vi "ChannelsHasWaveforms.vi"(11 "channels":T1[](array[typedef])) -> (2 "has waveforms":bool)   [LabVIEW 2017, in "DeviceModelHelpers.lvlib"]
doc: "Checks whether a channel has waveforms."
uses:
  <vilib>/addons/InsightCM/Utilities/DeviceModelHelpers/DeviceModelHelpers.lvlib
  <vilib>/addons/InsightCM/MessageBus/Base/controls/R2_Channel.ctl
  <vilib>/addons/InsightCM/MessageBus/Base/controls/KeyValuePair.ctl
  <vilib>/addons/InsightCM/MessageBus/Base/controls/Metric.ctl
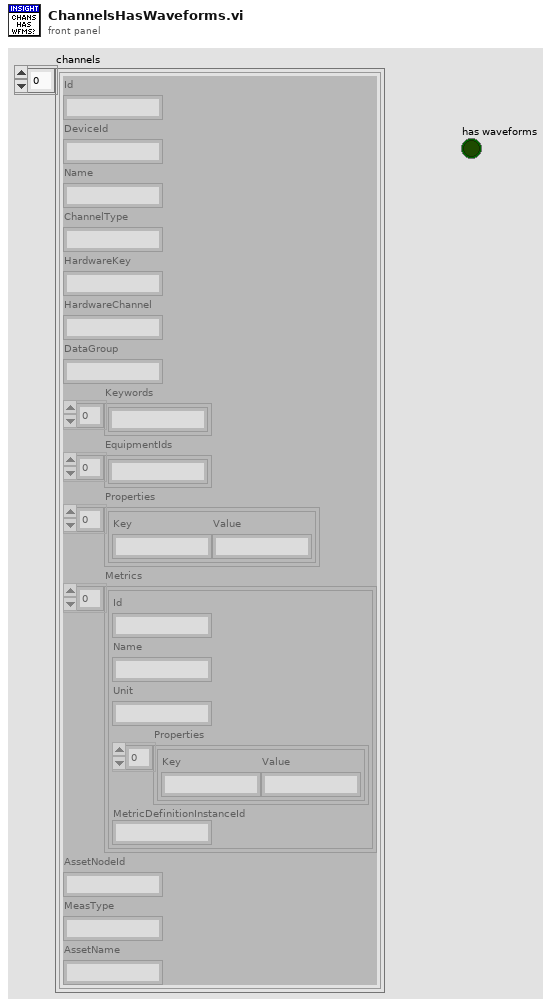
[diagram p1: front panel]
types:
  T1 = typedef "R2_Channel.ctl" = cluster{"Id":string, "DeviceId":string, "Name":string, "ChannelType":string, "HardwareKey":string, "HardwareChannel":string, "DataGroup":string, "Keywords":string[], "EquipmentIds":string[], "Properties":T2[], "Metrics":T3[], "AssetNodeId":string, "MeasType":string, "AssetName":string}
  T2 = typedef "KeyValuePair.ctl" = cluster{"Key":string, "Value":string}
  T3 = typedef "Metric.ctl" = cluster{"Id":string, "Name":string, "Unit":string, "Properties":T2[], "MetricDefinitionInstanceId":string}
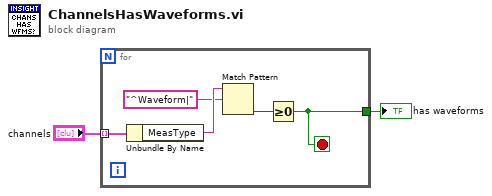
[diagram p0: block diagram]
diagram:
  n1 = for {
    tunnel: "channels" -> [w7] mode=indexing
    tunnel: [w3] -> w1
    stop <- w3 stop-if-true
    # "Search through each data group for waveforms; if none found, add to config"
    n2 = Unbundle By Name(w7) -> ("MeasType"=w6:string)
    n3 = Match Pattern(string=w6, regular expression="^Waveform|") -> (offset past match=w4:i32)  [unwired: 1 in, 3 out]
    n4 = Greater Or Equal To 0?(x=w4) -> (x >= 0?=w3:bool)
  }
  "has waveforms" <- w1
